vi "Momentary_Switch.vi"(9 "input_int":dbl, 10 "Type":T1(ring), 11 "input_bol":bool) -> (3 "out":bool)   [LabVIEW 2015]
panel:
  # "This subystem turns a button push into a momentary switch"
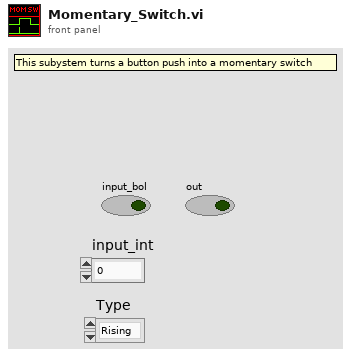
[diagram p1: front panel]
types:
  T1 = enum16{"Rising", "Falling", "Falling and Rising"}
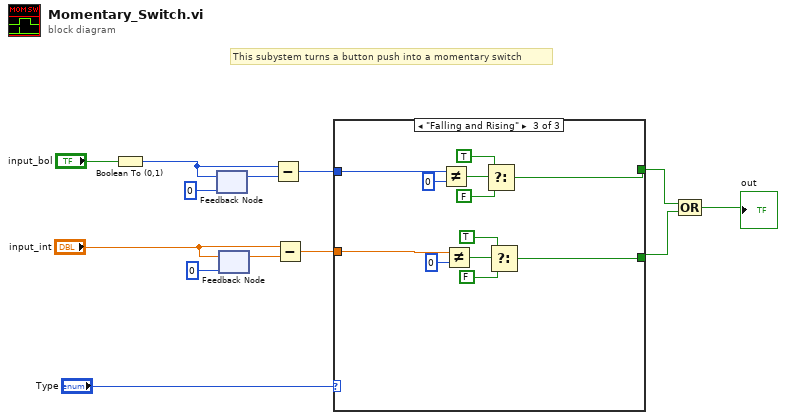
[diagram p0: block diagram]
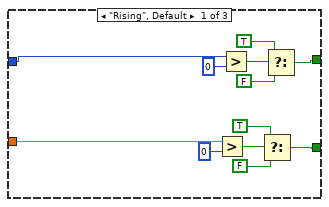
[diagram p2: hidden frame]
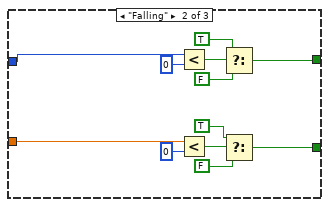
[diagram p3: hidden frame]
diagram:
  # "This subystem turns a button push into a momentary switch"
  n1 = Boolean To (0,1)(Boolean="input_bol") -> (0, 1=w8:i16)
  n2 = feedback #1(0) -> (w10:i32)
  n3 = feedback-in #1(w8) -> ()
  n4 = feedback #2(0) -> (w6:dbl)
  n5 = feedback-in #2("input_int") -> ()
  n6 = Subtract(x=w8, y=w10) -> (x-y=w9:i32)
  n7 = Subtract(x="input_int", y=w6) -> (x-y=w4:dbl)
  n8 = case shown="\"Falling and Rising\"" "Type" {
    tunnel: [w21 w37 w39] -> w3
    tunnel: w9 -> [w15 w28 w41]
    tunnel: w4 -> [w14 w27 w40]
    tunnel: [w16 w29 w38] -> w2
    frame "Rising", Default {
      n9 = Greater?(x=w14, y=0) -> (0:w19:bool)
      n10 = Greater?(x=w15, y=0) -> (0:w23:bool)
      n11 = Select(t=TRUE, s=w19, f=FALSE) -> (s? t:f=w16:bool)
      n12 = Select(t=TRUE, s=w23, f=FALSE) -> (s? t:f=w21:bool)
    }
    frame "Falling" {
      n13 = Less?(x=w28, y=0) -> (x < y?=w34:bool)
      n14 = Less?(x=w27, y=0) -> (x < y?=w31:bool)
      n15 = Select(t=TRUE, s=w34, f=FALSE) -> (s? t:f=w37:bool)
      n16 = Select(t=TRUE, s=w31, f=FALSE) -> (s? t:f=w29:bool)
    }
    frame "Falling and Rising" {
      n17 = Not Equal?(x=w41, y=0) -> (x != y?=w47:bool)
      n18 = Not Equal?(x=w40, y=0) -> (x != y?=w44:bool)
      n19 = Select(t=TRUE, s=w47, f=FALSE) -> (s? t:f=w39:bool)
      n20 = Select(t=TRUE, s=w44, f=FALSE) -> (s? t:f=w38:bool)
    }
  }
  n21 = Compound Arithmetic op=OR(w3, w2) -> (→"out":bool)
